vi "Show Front Panel Core.vi"(8 "error in (no error)":errorcluster, 10 "Data":T1, 11 "JQMHCore in":refnum<class "RQMHModule.lvclass">) -> (0 "error out":errorcluster, 3 "JQMHCore out":refnum<class "RQMHModule.lvclass">)   [LabVIEW 2024, in "RQMHModule.lvclass"]
uses:
  RQMHModule.lvclass
  Show Front Panel--Args.ctl
  RQMHModule.lvclass/RQMHModule.ctl
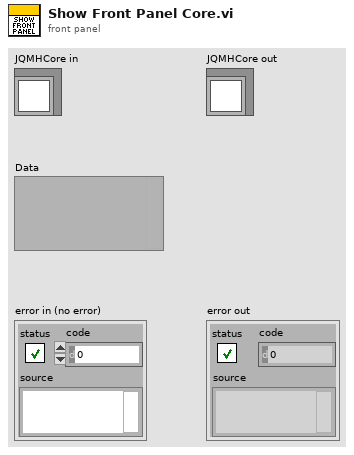
[diagram p1: front panel]
types:
  T1 = typedef "RQMHModule.lvclass/Show Front Panel--Args.ctl" = variant
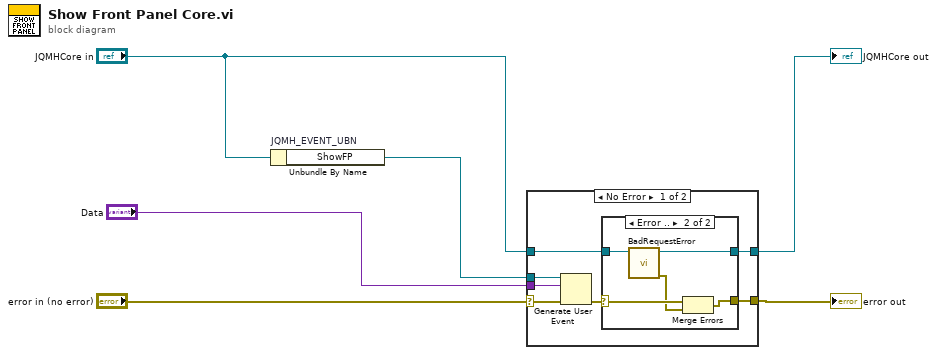
[diagram p0: block diagram]
diagram:
  n1 = Unbundle By Name "JQMH_EVENT_UBN"("JQMHCore in") -> ("ShowFP"=w6:refnum<user-event>)
  n2 = case shown="No Error" "error in (no error)" {
    selector: "error in (no error)" -> [w11 w21]
    tunnel: w6 -> [w13 _]
    tunnel: [w10 w21] -> w2
    tunnel: "JQMHCore in" -> [w8 w22]
    tunnel: [w9 w22] -> w5
    tunnel: "Data" -> [w7 _]
    frame No Error {
      n3 = Generate User Event(user event=w13, event data cluster=w7, error in=w11) -> (error out=w12:errorcluster)  [unwired: 1 in, 1 out]
      n4 = case shown="Error .." w12 {
        selector: w12 -> [w14 w20]
        tunnel: [w14 w19] -> w10
        tunnel: w8 -> [w15 w16]
        tunnel: [w15 w18] -> w9
        frame No Error {
        }
        frame Error {
          n5 = call "BadRequestError.vi"("JQMHModule in"=w16) -> ("error out"=w17:errorcluster, "JQMHModule out"=w18:refnum<class "RQMHModule.lvclass">)  [unwired: 9 in]
          n6 = Merge Errors(w20, w17) -> (w19:errorcluster)
        }
      }
    }
    frame Error {
    }
  }
  "error out" <- w2
  "JQMHCore out" <- w5
